vi "From JSON Text (U32).vi"(7 "Data Type (default value)":u32, 9 "error in (no error)":errorcluster, 10 "Offset":i32, 11 "JSON":string) -> (1 "error out":errorcluster, 2 "Offset past match":i32, 3 "Number":u32)   [LabVIEW 2017, in "JSONtext.lvlib"]
doc: "Convert the JSON Value at Offset into a LabVIEW type."
uses:
  JSONtext.lvlib
  support/Get U32.vi
  support/Get Number Text.vi
  Parsing/NaN or null to Integer ERROR.vi
  String Subset.vi
  Parsing/Advance past Number.vi
  support/Format Error.vi
  <vilib>/Utility/error.llb/Error Cluster From Error Code.vi
  Parsing/Parsing Error in converting to LabVIEW type.vi
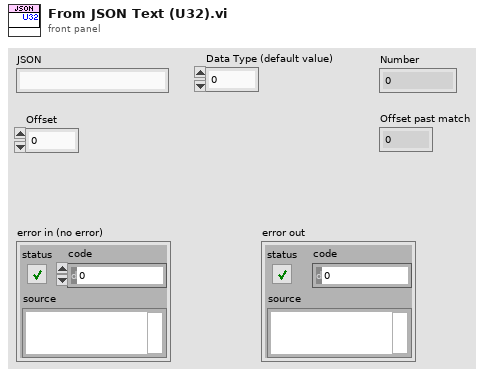
[diagram p1: front panel]
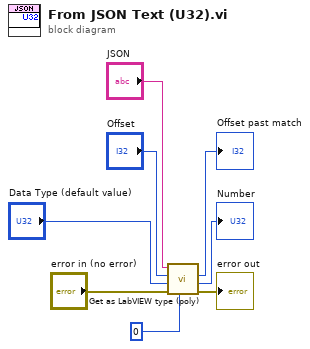
[diagram p0: block diagram]
diagram:
  n1 = call-poly "Get as LabVIEW type (poly).vi"("LV Type"=u32 0 ("Data Type (default value)"), "error in (no error)"="error in (no error)", "Data Type (default value)"="Data Type (default value)", "Offset"="Offset", "JSON"="JSON") -> ("error out"=→"error out":errorcluster, "Number"=→"Number":u32, "Offset past match"=→"Offset past match":i32)  [unwired: 4 in]
